vi "Modify_Indicies_of_Jumps_101+11_or_0_Case-1.vi"(3 "[IN] Subtracks":T1(array[cluster]), 4 "[IN] Indicies of sub\ntracks for transforma\ntion (resolving)":i32[](array[numeric]), 5 "[IN] Column Number":i32, 6 "[IN] Row Number":i32) -> (1 "[OUT] Indicies of Jumps":i32[](array[numeric]))   [LabVIEW 2013]
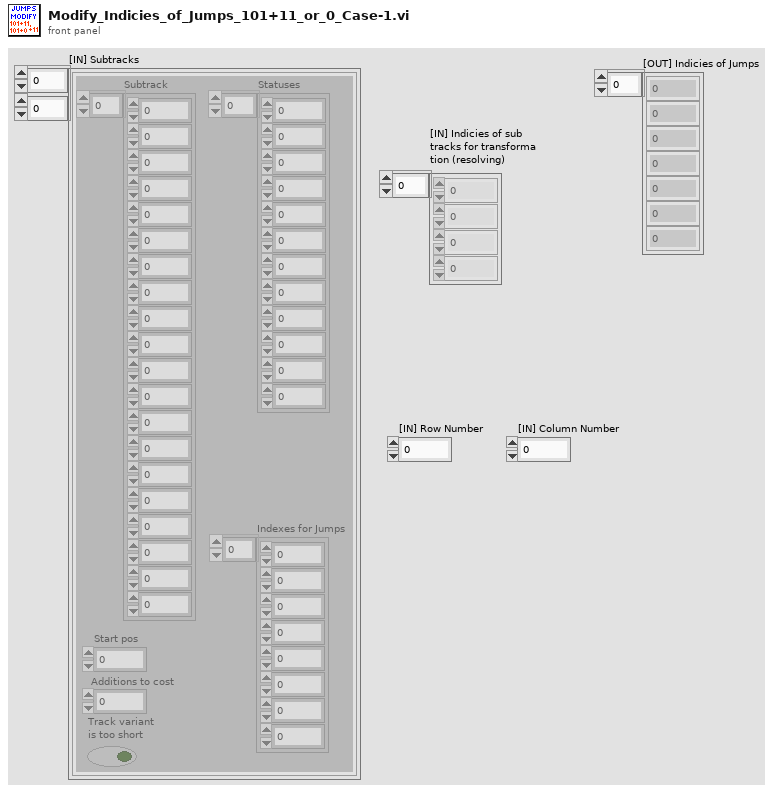
[diagram p1: front panel]
types:
  T1 = cluster{"Subtrack":dbl[], "Statuses":i16[], "Start pos":i32, "Additions to cost":i32, "Track variant \nis too short":bool, "Indexes for Jumps":i32[]}[][]
  T2 = cluster{"Subtrack":dbl[], "Statuses":i16[], "Start pos":i32, "Additions to cost":i32, "Track variant \nis too short":bool, "Indexes for Jumps":i32[]}
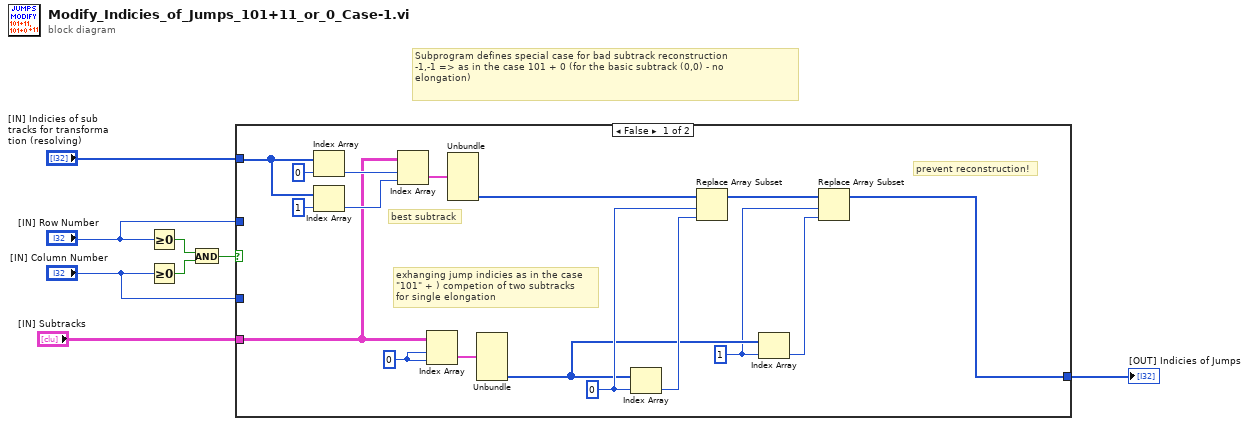
[diagram p0: block diagram]
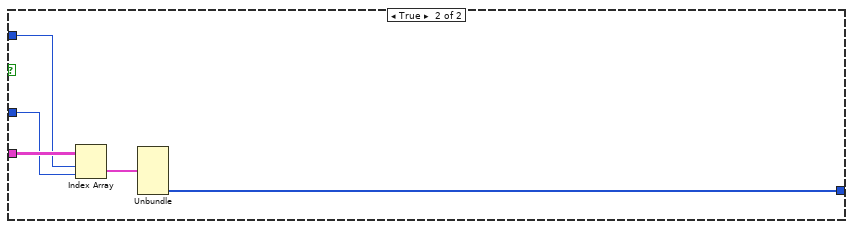
[diagram p2: hidden frame]
diagram:
  # "Subprogram defines special case for bad subtrack reconstruction\n-1,-1 => as in the case 101 + 0 (for the basic subtrack (0,0) - no \nelongation)"
  n1 = Greater Or Equal To 0?(x="[IN] Row Number") -> (x >= 0?=w6:bool)
  n2 = Greater Or Equal To 0?(x="[IN] Column Number") -> (x >= 0?=w5:bool)
  n3 = And(x=w6, y=w5) -> (x .and. y?=w4:bool)
  n4 = case shown="False" w4 {
    tunnel: "[IN] Indicies of sub\ntracks for transforma\ntion (resolving)" -> [w23 _]
    tunnel: "[IN] Subtracks" -> [w20 w30]
    tunnel: "[IN] Row Number" -> [_ w29]
    tunnel: "[IN] Column Number" -> [_ w28]
    tunnel: [w9 w26] -> w1
    frame False {
      w11 = 1 ("index")
      w15 = 0 ("index")
      w19 = 0 ("index (row)")
      # "prevent reconstruction!"
      # "best subtrack"
      # "exhanging jump indicies as in the case \n\"101\" + ) competion of two subtracks \nfor single elongation"
      n5 = Index Array(array=w23, index=0) -> (element=w22:i32)
      n6 = Index Array(array=w23, index=1) -> (element=w21:i32)
      n7 = Index Array(array=w20, index (row)=w22, index (col)=w21) -> (element=w18:T2)
      n8 = Index Array(array=w20, index (row)=w19, index (col)=w19) -> (element=w16:T2)
      n9 = Unbundle(w18) -> ("Indexes for Jumps"=w17:i32[])  [unwired: 5 out]
      n10 = Unbundle(w16) -> ("Indexes for Jumps"=w12:i32[])  [unwired: 5 out]
      n11 = Index Array(array=w12, index=w15) -> (element=w14:i32)
      n12 = Replace Array Subset(array=w17, new element=w14, index=w15) -> (w13:i32[])
      n13 = Index Array(array=w12, index=w11) -> (element=w10:i32)
      n14 = Replace Array Subset(array=w13, new element=w10, index=w11) -> (w9:i32[])
    }
    frame True {
      n15 = Index Array(array=w30, index (row)=w29, index (col)=w28) -> (element=w27:T2)
      n16 = Unbundle(w27) -> ("Indexes for Jumps"=w26:i32[])  [unwired: 5 out]
    }
  }
  "[OUT] Indicies of Jumps" <- w1
